vi "TagDB Table Probe.vi"(11 "DB Ref":refnum<k1>) -> (2 "Value String":string, 3 "Boolean":bool)   [LabVIEW 2017]
uses:
  <vilib>/Utility/Data Type/Type Definitions/Data Type.ctl
  <vilib>/Utility/Data Type/Type Definitions/Refnum Type.ctl
  <vilib>/Utility/Data Type/Type Definitions/VI Server Generic Type.ctl
  TagDB/_Support/Change Detector/TagDB dbChanged.vi
  dceec934-eb00-494d-a48d-fc1193159bd3.vi
  TagDB/_Support/DataAccess/TagDB Ref to DVR.vi
  TagDB/_Support/Error/_[error50000]Invalid DB REF.vi
  TagDB/_Support/Change Detector/TagDB ChangeFlag.vi
  TagDB/_Support/DataAccess/_NameCacher.vi
  TagDB/_Support/Error/_[error50002]Invalid DataType.vi
  TagDB/_Support/URL/TRIM-BOTH-SPACE.vi
  TagDB/_Support/Error/_Build Error Cluster.vi
  TagDB/TagDB.lvlib
  <vilib>/Utility/Data Type/NI_Data Type.lvlib
panel:
  out "Valid?":bool
  out "Name":string
  out "Last Item Change":timestamp format="%<%.3X>T"
  out "Last Data Change":timestamp format="%<%.3X>T"
  out "Array":T4(array[cluster])
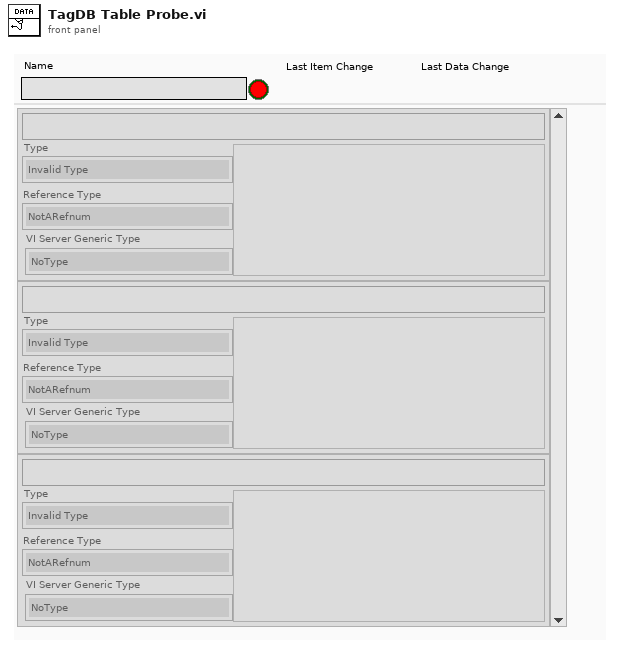
[diagram p1: front panel]
types:
  T1 = typedef "NI_Data Type.lvlib/Data Type.ctl" = enum8{"Invalid Type", "Void", "I8", "I16", "I32", "I64", "U8", "U16", "U32", "U64", "Single Float", "Double Float", "Extended Float", "Single Complex", "Double Complex", "Extended Complex", "Enum U8", "Enum U16", "Enum U32", "Enum U64", "Single Float With Unit", "Double Float With Unit", "Extended Float With Unit", "Single Complex with Unit", "Double Complex with Unit", "Extended Complex with Unit", "Boolean", "String", "Path", "Picture", "Tag", "Array", "Cluster", "Variant", "LV Variant", "Waveform", "Timestamp", "Digital Waveform", "Digital Data", "ExpressData", "Refnum", "External Data", "VI", "Poly VI", "LabVIEW Class Instance", "Fixed Point"}
  T2 = typedef "NI_Data Type.lvlib/Refnum Type.ctl" = enum16{"NotARefnum", "UnknownRefnum", "Generic", "Datalog", "ByteStream", "Device", "Occurence", "TCPNetConnection", "Auto", "Menu", "Imaq", "Hardware", "DataSocket", "Visa", "IVI", "UDPNetConnection", "Notifier", "Queue", "Irda", "EventReg", "DotNet", "UserEvent", "Callback", "UNUSED_EMPTY_POSITION", "BlueToothNetConnection", "LVObjApp", "LVObjVI", "LVObjUnknown", "GenericClass", "UserDefinedRefnumTag", "DataValue", "RT FIFO", "TDMS File"}
  T3 = typedef "NI_Data Type.lvlib/VI Server Generic Type.ctl" = enum16{"NoType", "\tkLVObjApp=0x1", "\tkLVObjVI", "\tkLVObjGeneric", "\tkLVObjDecoration", "\tkLVObjText", "\tkLVObjControl", "\tkLVObjColorBox", "\tkLVObjBoolean", "\tkLVObjRefNum", "\tkLVObjVariant", "\tkLVObjPath", "\tkLVObjListBox", "\tkLVObjTable", "\tkLVObjArray", "\tkLVObjPicture", "\tkLVObjOleContainer", "\tkLVObjNumeric", "\tkLVObjDigital", "\tkLVObjNamedNumeric", "\tkLVObjColorRamp", "\tkLVObjSlide", "\tkLVObjGraphOrChart", "\tkLVObjWaveformChart", "\tkLVObjWaveformGraph", "\tkLVObjIntensityChart", "\tkLVObjIntensityGraph", "\tkLVObjString", "\tkLVObjIOName", "\tkLVObjComboBox", "\tkLVObjCluster", "\tkLVObjPanel", "\tkLVObjKnob", "\tkLVObjNumWithScale", "\tkLVObjRing", "\tkLVObjEnum", "\tkLVObjGObject", "\tkLVObjPlot", "\tkLVObjCursor", "\tkLVObjNumericText", "\tkLVObjScale", "\tkLVObjColorScale", "\tkLVObjGraphScale", "\tkLVObjColorGraphScale", "\tkLVObjTypedRefNum", "\tkLVObjOldKnobScale", "\tkLVObjMCListbox", "\tkLVObjMeasureData", "\tkLVObjDSCTag", "\tkLVObjDAQName", "\tkLVObjVISAName", "\tkLVObjIVIName", "\tkLVObjSlideScale", "\tkLVObjTabControl", "\tkLVObjPage", "\tkLVObjTabArrayTabControl", "\tkLVObjConPane", "\tkLVObjDAQMXName", "\tkLVObjVIRefNum", "\tkLVObjLVObjRefNum", "\tkLVObjAbsTime", "\tkLVObjDigitalTable", "\tkLVObjUnused", "\tkLVObjUnused2", "\tkLVObjSCLControl", "\tkLVObjSubPanel", "\tkLVObjTreeControl", "\tkLVObjGenClassTagRef", "\tkLVObjGenClassRef", "\tkLVObjRotaryColorScale", "\tkLVObjPlugInDDOControl", "\tkLVObjPlugInDDOClassHolder", "\tkLVObjRadClusControl", "\tkLVObjProject", "\tkLVObjProjectItem", "\tkLVObjPane", "\tkLVObjSplitterBar", "\tkLVObjProjectBuildItem", "\tkLVObjPixmap", "\tkLVObjFacadeVI", "\tkLVObjLibrary", "\tkLVObjVariable", "\tkLVObjPropertyBag", "\tkLVObjXYGraph", "\tkLVObjScene", "\tkLVObjUDClassLibrary", "\tkLVObjUDClassClone", "\tkLVObjMethodVI", "\tkLVObjXCtlLibrary", "\tkLVObjXNodeLibrary", "\tkLVObjScroll", "\tkLVObjLVTarget", "\tkLVObjMixedGraph", "\tkLVObjProvider", "\tkLVObjCopyOperation", "\tkLVObjTargetItem", "\tkLVObjProjectItemType", "\tkLVObjCopyItem", "\tkLVObjCopyConflict", "\tkLVObjCopyExpert", "\tkLVObjSceneGraphDisp", "\tkLVObjPolyVI", "\tkLVObjLVClassDDO", "kLVObjDiagram=0x4000", "\tkLVObjTerminal", "\tkLVObjConstant", "\tkLVObjPathConstant", "\tkLVObjArrayConstant", "\tkLVObjNumericConstant", "\tkLVObjDigitalNumConstant", "\tkLVObjNamedNumericConstant", "\tkLVObjStringConstant", "\tkLVObjClusterConstant", "\tkLVObjFixedConstant", "\tkLVObjControlTerminal", "\tkLVObjFormulaParameter", "\tkLVObjGlobal", "\tkLVObjLocal", "\tkLVObjRightShiftRegister", "\tkLVObjFunction", "\tkLVObjSubVI", "\tkLVObjCallByRef", "\tkLVObjUnitCast", "\tkLVObjStructure", "\tkLVObjLoop", "\tkLVObjMultiframeStructure", "\tkLVObjSequence", "\tkLVObjCaseSelector", "\tkLVObjFormula", "\tkLVObjGrowableFunction", "\tkLVObjBuildClusterArray", "\tkLVObjCompoundArithmetic", "\tkLVObjIndexArray", "\tkLVObjBuildArray", "\tkLVObjNamedBundler", "\tkLVObjCIN", "\tkLVObjCallLibrary", "\tkLVObjObjectFunction", "\tkLVObjProperty", "\tkLVObjInvoke", "\tkLVObjNode", "\tkLVObjBooleanConstant", "\tkLVObjBlockDiagram", "\tkLVObjRingConstant", "\tkLVObjEnumConstant", "\tkLVObjTunnel", "\tkLVObjLoopTunnel", "\tkLVObjSequenceLocal", "\tkLVObjComparison", "\tkLVObjReadWriteFile", "\tkLVObjTypeCast", "\tkLVObjFlattenUnflattenString", "\tkLVObjGPIBReadWrite", "\tkLVObjForLoop", "\tkLVObjWhileLoop", "\tkLVObjScriptNode", "\tkLVObjArrayToCluster", "\tkLVObjFormatScanString", "\tkLVObjWire", "\tkLVObjProbe", "\tkLVObjInnerTerminal", "\tkLVObjLeftShiftRegister", "\tkLVObjPolySubVI", "\tkLVObjPropItem", "\tkLVObjIONameConstant", "\tkLVObjDSCTagConstant", "\tkLVObjDAQNameConstant", "\tkLVObjVISANameConstant", "\tkLVObjIVINameConstant", "\tkLVObjColorBoxConstant", "\tkLVObjControlRefConstant", "\tkLVObjClassSpecifierConstant", "\tkLVObjConfNode", "\tkLVObjMasterWizard", "\tkLVObjStateDiagWizard", "\tkLVObjOuterTerminal", "\tkLVObjDAQMXNameConstant", "\tkLVObjEventStructure", "\tkLVObjFlatSequence", "\tkLVObjGenClassTagRefConstant", "\tkLVObjAbsTimeConstant", "\tkLVObjExternalNode", "\tkLVObjSubWizard", "\tkLVObjScriptNodeParameter", "\tkLVObjStatVIRef", "\tkLVObjComboBoxConstant", "\tkLVObjTimedLoop", "\tkLVObjGenClassDeepCopy", "\tkLVObjGenClassTagFlat", "\tkLVObjGenClassTagFlatRefConstant", "\tkLVObjGenClassFlat", "\tkLVObjSimDiagram", "\tkLVObjCompDiagram", "\tkLVObjSimNode", "\tkLVObjSimDCO", "\tkLVObjBundler", "\tkLVObjUnbundler", "\tkLVObjNamedUnbundler", "\tkLVObjFlatSeqFrame", "\tkLVObjFlatSeqInTun", "\tkLVObjFlatSeqOutTun", "\tkLVObjRefNumConst", "\tkLVObjFlattenString", "\tkLVObjPolySelector", "\tkLVObjXNode", "\tkLVObjSelectorTunnel", "\tkLVObjCommentNode", "\tkLVObjSdfDiagram", "\tkLVObjSDFCompDiagram", "\tkLVObjSdfNode", "\tkLVObjSdfDCO", "\tkLVObjFileDialog", "\tkLVObjTLDCO", "\tkLVObjTimeSeqFrame", "\tkLVObjTimeFlatSequence", "\tkLVObjTimedSequence", "\tkLVObjXDataNode", "\tkLVObjCodeWizard", "\tkLVObjMathScriptNode", "\tkLVObjMathScriptNodeParameter", "\tkLVObjLVClassBDConst"}
  T4 = cluster{"Tag":string, "Type":T1, "Reference Type":T2, "VI Server Generic Type":T3, "Value":variant}[]
  T5 = enum8{"Enabled", "Disabled", "Disabled and Grayed Out"}
  T6 = cluster{"ClassName":string, "Reference":refnum<vi>}
  T7 = cluster{string, "Type":T1, "Reference Type":T2, "VI Server Generic Type":T3, "Variant":variant}
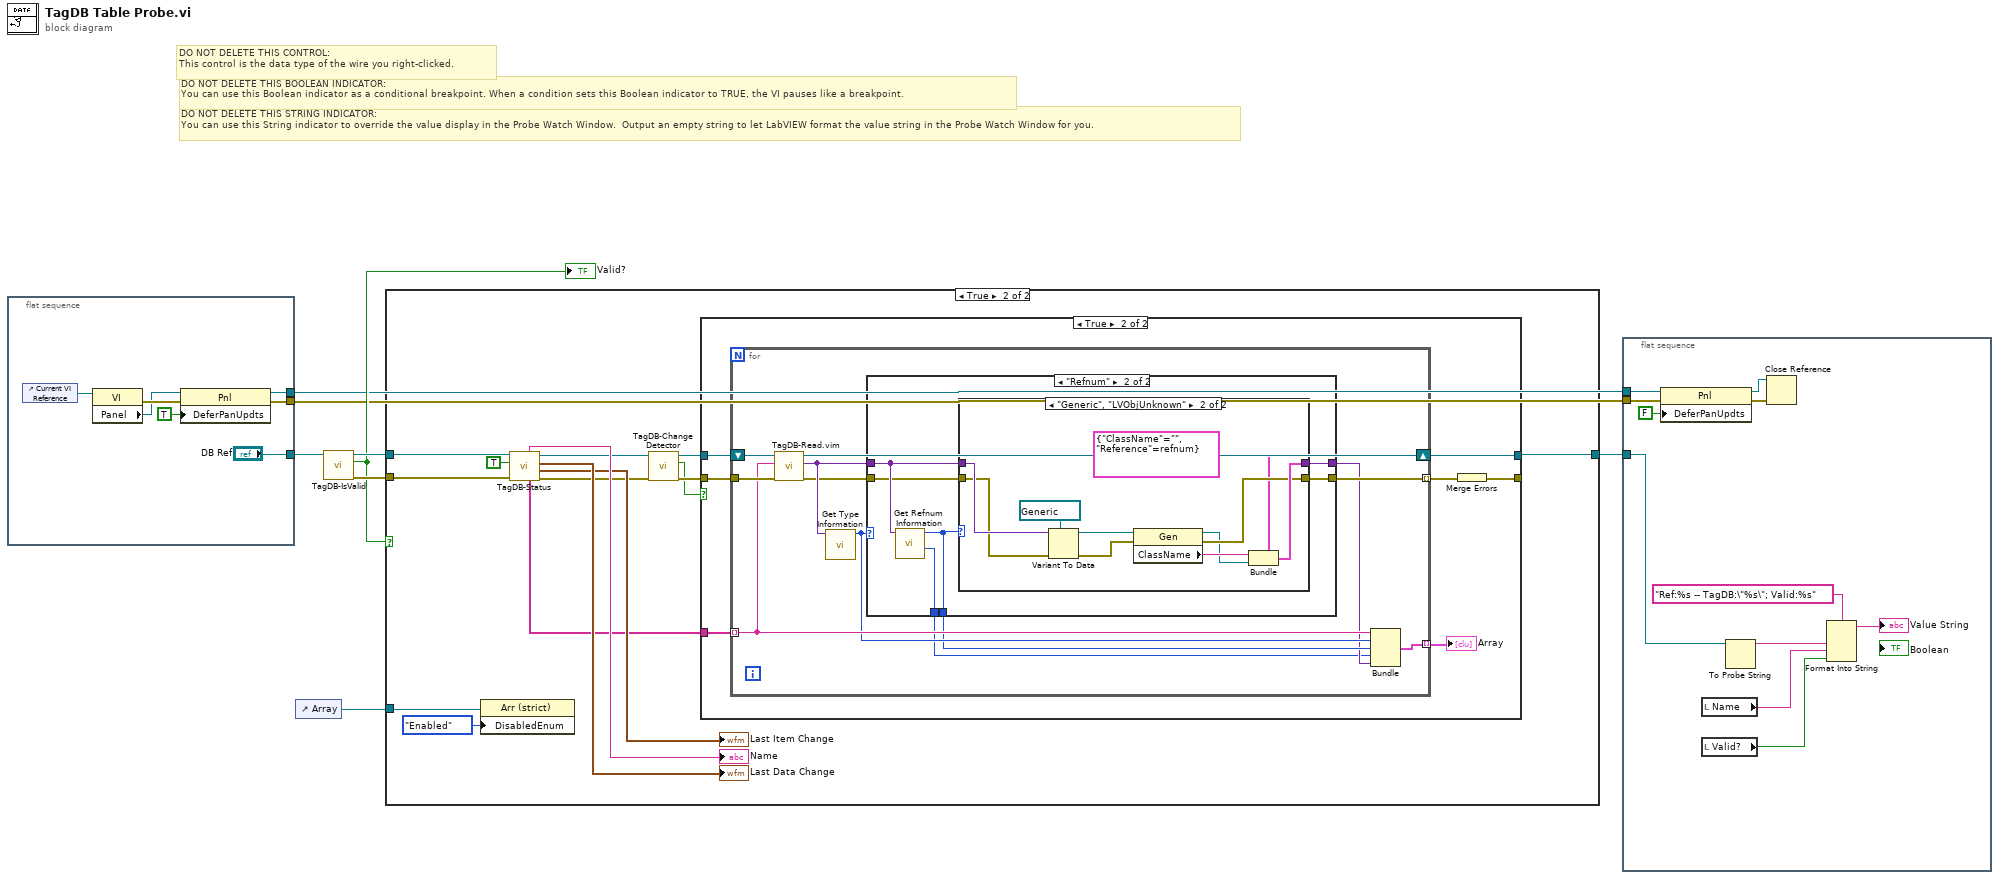
[diagram p0: block diagram]
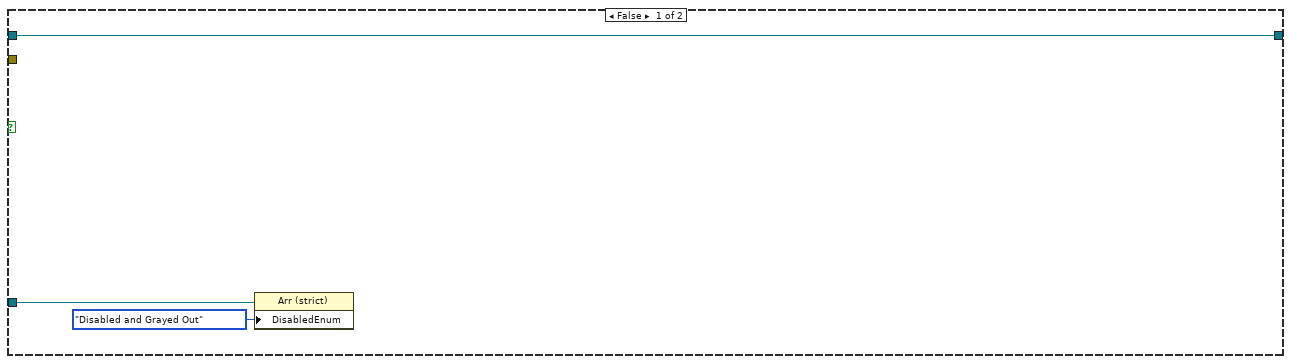
[diagram p2: hidden frame]
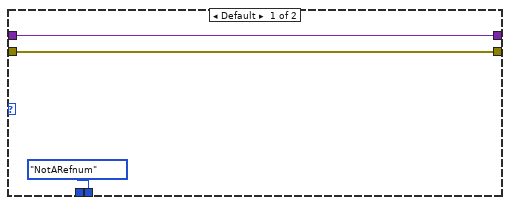
[diagram p4: hidden frame]
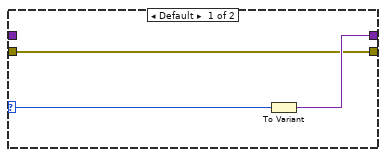
[diagram p5: hidden frame]
diagram:
  # "DO NOT DELETE THIS STRING INDICATOR: \nYou can use this String indicator to override the value display in the Probe Watch Window.  Output an empty string to let LabVIEW format the value string in the Probe Watch Window for you."
  # "DO NOT DELETE THIS BOOLEAN INDICATOR: \nYou can use this Boolean indicator as a conditional breakpoint. When a condition sets this Boolean indicator to TRUE, the VI pauses like a breakpoint."
  # "DO NOT DELETE THIS CONTROL: \nThis control is the data type of the wire you right-clicked."
  n1 = flat-sequence {
    tunnel: [w11] -> w2
    tunnel: [w10] -> w3
    tunnel: ["DB Ref"] -> w4
    frame #0 {
      n2 = control-ref of="Current VI Reference"() -> (w15:refnum<vi>)
      n3 = property class="VI"(reference=w15) -> (error out=w14:errorcluster, "Panel"=w13:refnum<vi>)  [unwired: 1 in, 1 out]
      n4 = property class="Pnl"(reference=w13, error in=w14, "DeferPanUpdts"=TRUE ("Defer Panel Updates")) -> (reference out=w11:refnum<vi>, error out=w10:errorcluster)
    }
  }
  n5 = control-ref of="Array"() -> (w5:refnum<vi>)
  n6 = call "TagDB-IsValid.vi"("TagDB"=w4) -> ("error out"=w7:errorcluster, "valid TagDB?"=w6:bool, "TagDB(dup)"=w8:refnum<k1>)  [unwired: 8 in]
  "Valid?" <- w6
  n7 = case shown="True" w6 {
    tunnel: w8 -> [w16 w33]
    tunnel: w7 -> [_ w32]
    tunnel: w5 -> [w17 w20]
    tunnel: [w16 w19] -> w1
    frame False {
      n8 = property class="Arr (strict)"(reference=w17, "DisabledEnum"=T5."Disabled and Grayed Out" ("Disabled")) -> ()  [unwired: 1 in, 2 out]
    }
    frame True {
      n9 = property class="Arr (strict)"(reference=w20, "DisabledEnum"=T5."Enabled" ("Disabled")) -> ()  [unwired: 1 in, 2 out]
      n10 = call "TagDB-Status.vi"("error in (no error)"=w32, "return elements? (F)"=TRUE, "DB Ref"=w33) -> ("error out"=w24:errorcluster, "Item Change Timestamp"=→"Last Item Change":timestamp, "Global Change Timestamp"=→"Last Data Change":timestamp, "DB Ref(dup)"=w25:refnum<k1>, "DB items"=w22:string[], "db name"=→"Name":string)  [unwired: 3 in]
      n11 = call-poly "TagDB-Change Detector.vi"("error in (no error)"=w24, "DB Ref"=w25) -> ("error in (no error) (dup)"=w27:errorcluster, "changed?"=w26:bool, "DB Ref (dup)"=w28:refnum<k1>)  [unwired: 7 in]
      n12 = case shown="True" w26 {
        tunnel: [w35 w42] -> w19
        tunnel: [w34 w36] -> _
        tunnel: w22 -> [_ w40]
        tunnel: w28 -> [w35 w39]
        tunnel: w27 -> [w34 w38]
        frame False {
        }
        frame True {
          n13 = for {
            tunnel: w40 -> [w48] mode=indexing
            shift-right: [w53] -> w42
            shift-left: w39 -> [w54]
            tunnel: [w44] -> w37 mode=indexing
            tunnel: w38 -> [w51]
            tunnel: [w52] -> w41 mode=indexing
            n14 = call "TagDB-Read.vim"("error in (no error)"=w51, "name"=w48, "TagDB"=w54) -> ("error out"=w49:errorcluster, "Value"=w50:variant, "TagDB(dup)"=w53:refnum<k1>)  [unwired: 3 in, 3 out]
            n15 = call <vilib>:"Get Type Information.vi"("Variant"=w50) -> ("Type"=w47:T1)  [unwired: 6 in, 4 out]
            n16 = case shown="\"Refnum\"" w47 {
              tunnel: [w57 w63] -> w45
              tunnel: w50 -> [w57 w62]
              tunnel: w49 -> [w56 w61]
              tunnel: [w56 w60] -> w52
              tunnel: [Refnum_Type."NotARefnum" ("Reference Type") w59] -> w46
              tunnel: [_ w58] -> w43
              frame Default {
              }
              frame "Refnum" {
                n17 = call <vilib>:"Get Refnum Information.vi"("Variant"=w62) -> ("VI Server Generic Type"=w58:T3, "Reference Type"=w59:T2)  [unwired: 7 in, 2 out]
                n18 = case shown="\"Generic\", \"LVObjUnknown\"" w59 {
                  selector: w59 -> [w66 _]
                  tunnel: [w65 w73] -> w63
                  tunnel: w62 -> [_ w76]
                  tunnel: w61 -> [w64 w72]
                  tunnel: [w64 w71] -> w60
                  frame Default {
                    n19 = To Variant(anything=w66) -> (Variant=w65:variant)
                  }
                  frame "Generic", "LVObjUnknown" {
                    n20 = Variant To Data(error in=w72, type=refnum<vi> refnum ("value"), Variant=w76) -> (data=w74:refnum<vi>, error out=w69:errorcluster)
                    n21 = property class="Gen"(reference=w74, error in=w69) -> (reference out=w67:refnum<vi>, error out=w71:errorcluster, "ClassName"=w68:string)
                    n22 = Bundle(cluster=T6 {"ClassName"="", "Reference"=refnum}, "ClassName"=w68, "Reference"=w67) -> (w73:T6)
                  }
                }
              }
            }
            n23 = Bundle(w48, "Type"=w47, "Reference Type"=w46, "VI Server Generic Type"=w43, "Variant"=w45) -> (w44:T7)  [unwired: 1 in]
          }
          "Array" <- w37
          n24 = Merge Errors(w41) -> (w36:errorcluster)
        }
      }
    }
  }
  n25 = flat-sequence {
    tunnel: w2 -> [w86]
    tunnel: w3 -> [w85]
    tunnel: w1 -> [w80]
    frame #0 {
      n26 = property class="Pnl"(reference=w86, error in=w85, "DeferPanUpdts"=FALSE ("Defer Panel Updates")) -> (reference out=w83:refnum<vi>, error out=w84:errorcluster)
      n27 = local read "Name"() -> (w78:string)
      n28 = local read "Valid?"() -> (w77:bool)
      n29 = To Probe String(7:w80) -> (3:w81:string)  [unwired: 2 in, 1 out]
      n30 = Close Reference(reference=w83, error in (no error)=w84) -> ()  [unwired: 1 out]
      n31 = Format Into String(format string="Ref:%s -- TagDB:\"%s\"; Valid:%s", w81, w78, w77) -> (resulting string=→"Value String":string)  [unwired: 2 in, 1 out]
    }
  }
